vi "Update FP.vi"(5 "update picture (T)":bool=TRUE, 7 "FP refs":T2, 8 "error in (no error)":errorcluster, 9 "data row index":i32, 10 "rangefinder data in":T1, 11 "draw options in":T3={"Background Color"=16777215, "Grid Color"=13816530, "Angle Units"=enum."Radians", "Draw Solid Background"=TRUE, "Draw Grid"=TRUE, "Grid Spacing"=1.0, "AutoScale"=TRUE, "Fit to Radius"=1.0, "data row options"=[]}) -> (0 "error out":errorcluster, 2 "rangefinder data out":T1, 3 "draw options out":T3={"Background Color"=16777215, "Grid Color"=13816530, "Angle Units"=enum."Radians", "Draw Solid Background"=TRUE, "Draw Grid"=TRUE, "Grid Spacing"=1.0, "AutoScale"=TRUE, "Fit to Radius"=1.0, "data row options"=[]})   [LabVIEW 2017, in "NI_Robotics_2D Rangefinder.xctl" / "Config Dialog.lvlib"]
uses:
  <vilib>/robotics/Controls/2D Rangefinder/_2D Rangefinder Support Files/Configuration/Config Dialog.lvlib
  <vilib>/robotics/Controls/2D Rangefinder/2D Rangefinder Picture/Draw Options.ctl
  <vilib>/robotics/Controls/Utilities/Angle Units.ctl
  <vilib>/robotics/Controls/2D Rangefinder/2D Rangefinder Picture/Data Row Options.ctl
  <vilib>/robotics/Controls/2D Rangefinder/_2D Rangefinder Support Files/Configuration/FP Refs.ctl
  <vilib>/robotics/Controls/2D Rangefinder/2D Rangefinder Picture/Rangefinder Data.ctl
  <vilib>/robotics/Controls/2D Rangefinder/2D Rangefinder Picture/NI_Robotics_2D Rangefinder Picture.lvlib
  <vilib>/robotics/Controls/Utilities/NI_Robotics_Control Utilities.lvlib
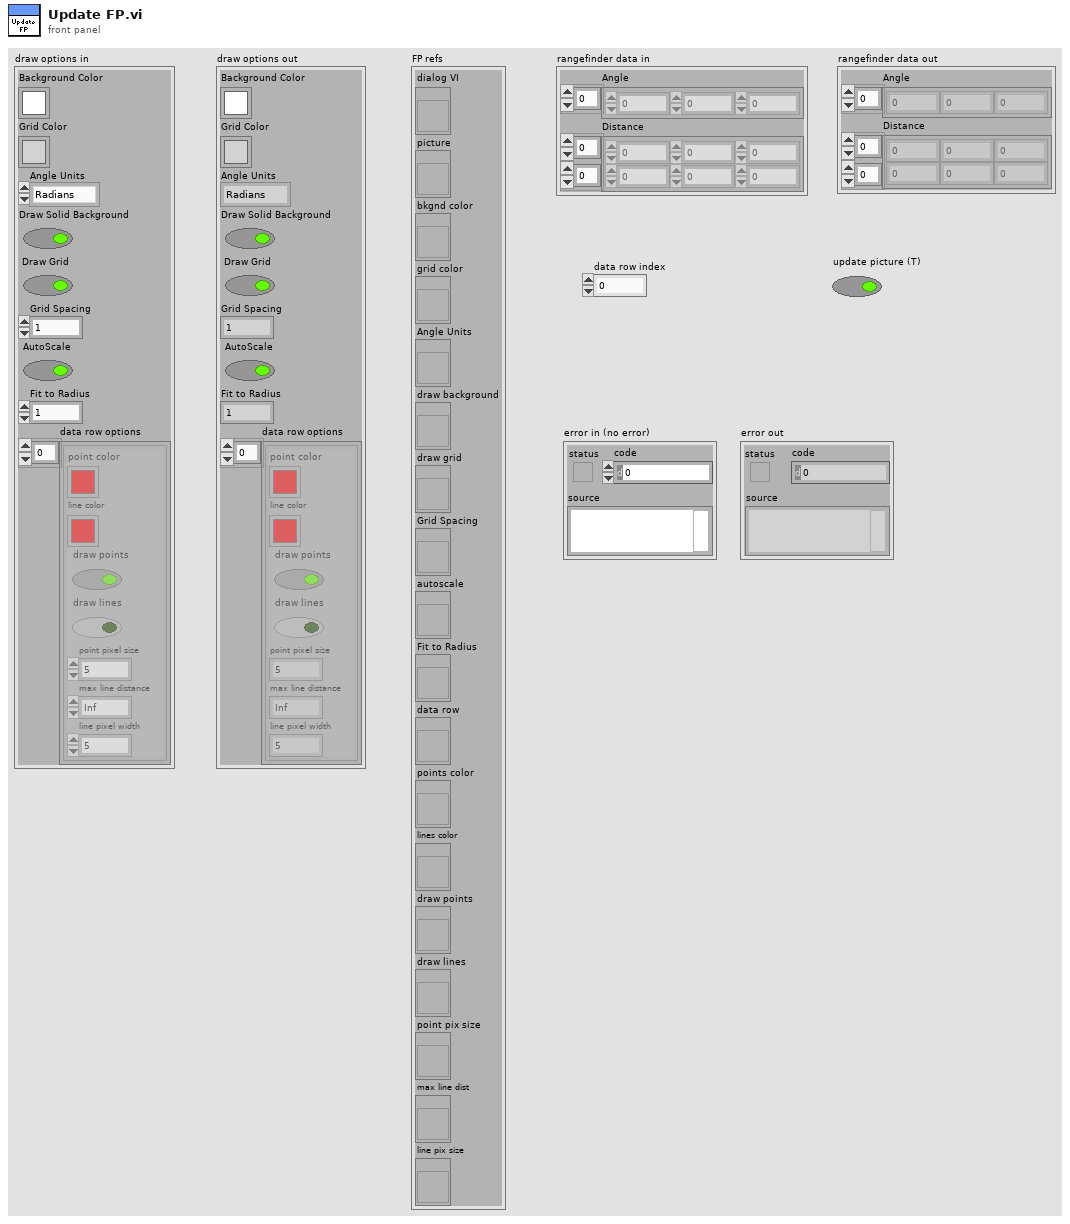
[diagram p1: front panel]
types:
  T1 = typedef "NI_Robotics_2D Rangefinder Picture.lvlib/Rangefinder Data.ctl" = cluster{"Angle":dbl[], "Distance":dbl[][]}
  T2 = typedef "NI_Robotics_2D Rangefinder.xctl/Config Dialog.lvlib/FP Refs.ctl" = cluster{"dialog VI":refnum<vi>, "picture":refnum<vi>, "bkgnd color":refnum<vi>, "grid color":refnum<vi>, "Angle Units":refnum<vi>, "draw background":refnum<vi>, "draw grid":refnum<vi>, "Grid Spacing":refnum<vi>, "autoscale":refnum<vi>, "Fit to Radius":refnum<vi>, "data row":refnum<vi>, "points color":refnum<vi>, "lines color":refnum<vi>, "draw points":refnum<vi>, "draw lines":refnum<vi>, "point pix size":refnum<vi>, "max line dist":refnum<vi>, "line pix size":refnum<vi>}
  T3 = typedef "NI_Robotics_2D Rangefinder Picture.lvlib/Draw Options.ctl" = cluster{"Background Color":u32, "Grid Color":u32, "Angle Units":T4, "Draw Solid Background":bool, "Draw Grid":bool, "Grid Spacing":dbl, "AutoScale":bool, "Fit to Radius":dbl, "data row options":T5[]}
  T4 = typedef "NI_Robotics_Control Utilities.lvlib/Angle Units.ctl" = enum16{"Radians", "Degrees"}
  T5 = typedef "NI_Robotics_2D Rangefinder Picture.lvlib/Data Row Options.ctl" = cluster{"point color":u32, "line color":u32, "draw points":bool, "draw lines":bool, "point pixel size":u16, "max line distance":dbl, "line pixel width":u16}
  T6 = typedef "LVBoundsTypeDef.ctl" = cluster{"Width":u32, "Height":u32}
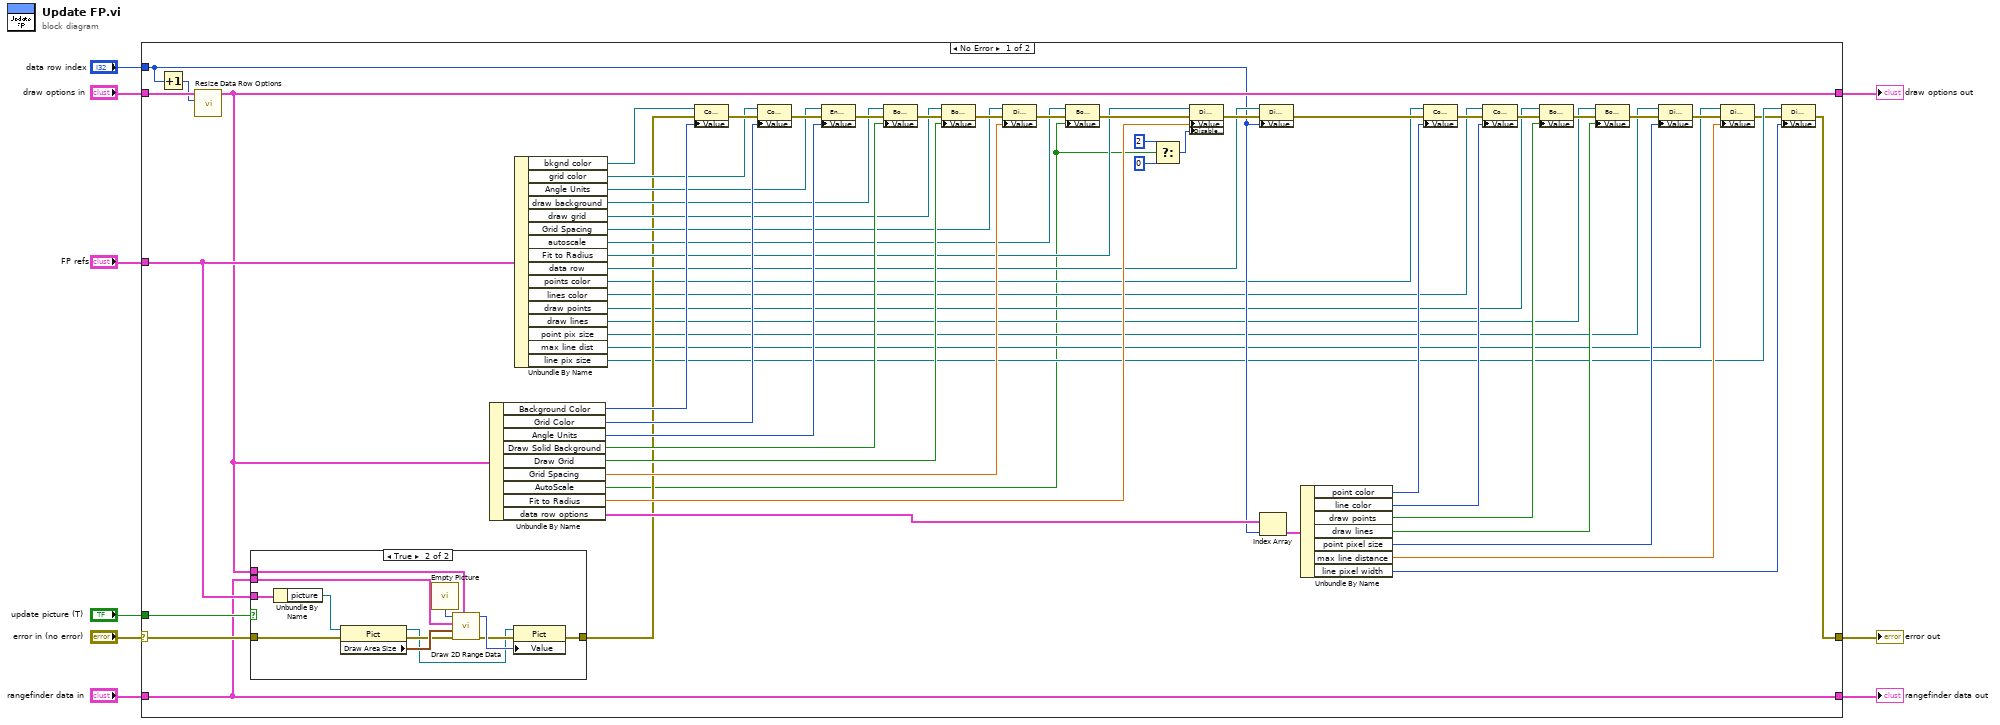
[diagram p0: block diagram]
diagram:
  n1 = case shown="No Error" "error in (no error)" {
    selector: "error in (no error)" -> [w69 w86]
    tunnel: [w15 w86] -> w8
    tunnel: "FP refs" -> [w68 _]
    tunnel: "update picture (T)" -> [w70 _]
    tunnel: "draw options in" -> [w43 w85]
    tunnel: "rangefinder data in" -> [w14 w84]
    tunnel: [w41 w85] -> w3
    tunnel: [w14 w84] -> w2
    tunnel: "data row index" -> [w38 _]
    frame No Error {
      n2 = Increment(x=w38) -> (x+1=w42:i32)
      n3 = call <vilib>:"Resize Data Row Options.vi"("number of data rows (1)"=w42, "draw options in"=w43) -> ("draw options out"=w41:T3)  [unwired: 9 in]
      n4 = case shown="True" w70 {
        tunnel: w68 -> [_ w83]
        tunnel: w41 -> [_ w81]
        tunnel: w69 -> [w71 w77]
        tunnel: w14 -> [_ w76]
        tunnel: [w71 w73] -> w37
        frame False {
        }
        frame True {
          n5 = Unbundle By Name(w83) -> ("picture"=w78:refnum<vi>)
          n6 = property class="Pict"(reference=w78, error in=w77) -> (reference out=w72:refnum<vi>, error out=w79:errorcluster, "Draw Area Size"=w80:T6)
          n7 = call "Empty Picture"() -> ("empty picture"=w82:picture)
          n8 = call <vilib>:"Draw 2D Range Data.vi"("draw options"=w81, "error in (no error)"=w79, "DrawAreaSize"=w80, "data"=w76, "picture in"=w82) -> ("error out"=w74:errorcluster, "picture out"=w75:picture)  [unwired: 5 in]
          n9 = property class="Pict"(reference=w72, error in=w74, "Value"=w75) -> (error out=w73:errorcluster)  [unwired: 1 out]
        }
      }
      n10 = Unbundle By Name(w41) -> ("Background Color"=w64:u32, "Grid Color"=w61:u32, "Angle Units"=w58:T4, "Draw Solid Background"=w55:bool, "Draw Grid"=w52:bool, "Grid Spacing"=w49:dbl, "AutoScale"=w13:bool, "Fit to Radius"=w44:dbl, "data row options"=w67:T5[])
      n11 = Unbundle By Name(w68) -> ("bkgnd color"=w65:refnum<vi>, "grid color"=w62:refnum<vi>, "Angle Units"=w59:refnum<vi>, "draw background"=w56:refnum<vi>, "draw grid"=w53:refnum<vi>, "Grid Spacing"=w50:refnum<vi>, "autoscale"=w47:refnum<vi>, "Fit to Radius"=w45:refnum<vi>, "data row"=w39:refnum<vi>, "points color"=w35:refnum<vi>, "lines color"=w32:refnum<vi>, "draw points"=w29:refnum<vi>, "draw lines"=w26:refnum<vi>, "point pix size"=w23:refnum<vi>, "max line dist"=w20:refnum<vi>, "line pix size"=w18:refnum<vi>)
      n12 = property class="ColBox"(reference=w65, error in=w37, "Value"=w64) -> (error out=w63:errorcluster)  [unwired: 1 out]
      n13 = property class="ColBox"(reference=w62, error in=w63, "Value"=w61) -> (error out=w60:errorcluster)  [unwired: 1 out]
      n14 = property class="Enum (strict)"(reference=w59, error in=w60, "Value"=w58) -> (error out=w57:errorcluster)  [unwired: 1 out]
      n15 = property class="Bool (strict)"(reference=w56, error in=w57, "Value"=w55) -> (error out=w54:errorcluster)  [unwired: 1 out]
      n16 = property class="Bool (strict)"(reference=w53, error in=w54, "Value"=w52) -> (error out=w51:errorcluster)  [unwired: 1 out]
      n17 = property class="DigNum (strict)"(reference=w50, error in=w51, "Value"=w49) -> (error out=w48:errorcluster)  [unwired: 1 out]
      n18 = property class="Bool (strict)"(reference=w47, error in=w48, "Value"=w13) -> (error out=w46:errorcluster)  [unwired: 1 out]
      n19 = Select(t=u8 2, s=w13, f=u8 0) -> (s? t:f=w10:u8)
      n20 = property class="DigNum (strict)"(reference=w45, error in=w46, "Value"=w44, "DisabledEnum"=w10) -> (error out=w40:errorcluster)  [unwired: 1 out]
      n21 = property class="DigNum (strict)"(reference=w39, error in=w40, "Value"=w38) -> (error out=w36:errorcluster)  [unwired: 1 out]
      n22 = Index Array(array=w67, index=w38) -> (element=w66:T5)
      n23 = Unbundle By Name(w66) -> ("point color"=w34:u32, "line color"=w31:u32, "draw points"=w28:bool, "draw lines"=w25:bool, "point pixel size"=w22:u16, "max line distance"=w19:dbl, "line pixel width"=w16:u16)
      n24 = property class="ColBox"(reference=w35, error in=w36, "Value"=w34) -> (error out=w33:errorcluster)  [unwired: 1 out]
      n25 = property class="ColBox"(reference=w32, error in=w33, "Value"=w31) -> (error out=w30:errorcluster)  [unwired: 1 out]
      n26 = property class="Bool (strict)"(reference=w29, error in=w30, "Value"=w28) -> (error out=w27:errorcluster)  [unwired: 1 out]
      n27 = property class="Bool (strict)"(reference=w26, error in=w27, "Value"=w25) -> (error out=w24:errorcluster)  [unwired: 1 out]
      n28 = property class="DigNum (strict)"(reference=w23, error in=w24, "Value"=w22) -> (error out=w21:errorcluster)  [unwired: 1 out]
      n29 = property class="DigNum (strict)"(reference=w20, error in=w21, "Value"=w19) -> (error out=w17:errorcluster)  [unwired: 1 out]
      n30 = property class="DigNum (strict)"(reference=w18, error in=w17, "Value"=w16) -> (error out=w15:errorcluster)  [unwired: 1 out]
    }
    frame Error {
    }
  }
  "draw options out" <- w3
  "error out" <- w8
  "rangefinder data out" <- w2
